vi "Get Sciscan GFG_core Reference.vi"(8 "error in":errorcluster, 11 "file path":path) -> (0 "error out":errorcluster, 1 "Sciscan Event":refnum<user-event>, 2 "RGB overlay":T1, 3 "GFG reference":refnum<vi>)   [LabVIEW 2012, in "Sciscan Scope Daemon.lvlib"]
uses:
  Sciscan Scope Daemon.lvlib
  <vilib>/vision/Image Controls.llb/IMAQ Image.ctl
  <vilib>/Utility/VariantDataType/Type.ctl
  <vilib>/Utility/VariantDataType/VariantType.lvlib
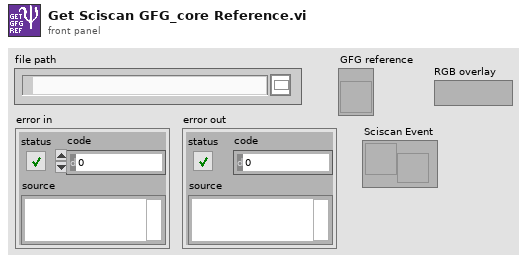
[diagram p1: front panel]
types:
  T1 = typedef "IMAQ Image.ctl" = refnum<image>
  T2 = enum16{"open", "replace", "create", "open or create", "replace or create", "replace or create with confirmation"}
  T3 = cluster{"Channel 1 small":T1, "Channel 2 small":T1, "Channel 3 small":T1, "Channel 4 small":T1, "Channel 1 large":T1, "Channel 2 large":T1, "Channel 3 large":T1, "Channel 4 large":T1, "RGB overlay":T1, "ROI Image display":T1, "arb line scan display":T1, "Channel 5 large":T1}
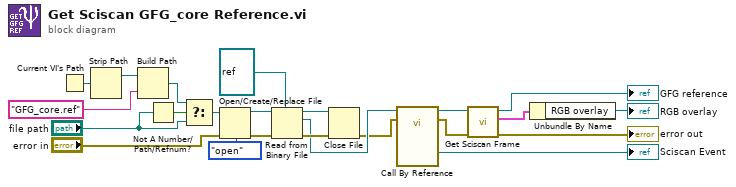
[diagram p0: block diagram]
diagram:
  n1 = Current VI's Path() -> (path=w18:path)
  n2 = Strip Path(path=w18) -> (stripped path=w17:path)  [unwired: 1 out]
  n3 = Build Path(base path=w17, name or relative path="GFG_core.ref" ("replace string (\"\")")) -> (appended path=w15:path)
  n4 = Not A Number/Path/Refnum?(number/path/refnum="file path") -> (NaN/Path/Refnum?=w13:bool)
  n5 = Select(t=w15, s=w13, f="file path") -> (s? t:f=w14:path)
  n6 = Open/Create/Replace File(file path (use dialog)=w14, error in="error in", operation (0:open)=T2."open") -> (refnum out=w21:refnum<file>, error out=w22:errorcluster)  [unwired: 3 in, 1 out]
  n7 = Read from Binary File(5:refnum<vi> refnum ("application reference (local)"), 8:w22, 11:w21) -> (0:w19:errorcluster, 2:w4:refnum<vi>, 3:w20:refnum<file>)  [unwired: 3 in, 1 out]
  n8 = Close File(refnum=w20, error in=w19) -> (error out=w3:errorcluster)  [unwired: 1 out]
  n9 = call-by-ref "?"(reference=w4, error in=w3) -> (reference out=w5:refnum<vi>, error out=w2:errorcluster, "user event out"=→"Sciscan Event":refnum<user-event>)  [unwired: 13 in, 6 out]
  n10 = call "Get Sciscan Frame.vi"("error in (no error)"=w2, "GFG reference"=w5) -> ("error out"=→"error out":errorcluster, "image refs out"=w9:T3, "GFG reference"=→"GFG reference":refnum<vi>)  [unwired: 7 in]
  n11 = Unbundle By Name(w9) -> ("RGB overlay"=→"RGB overlay":T1)
